vi "Distancias_ejes_convoy.vi"(2 "Series_flota1":string[](array[string]), 3 "Ejes_UT":i32[](array[numeric]), 4 "Puntos medios de las ventanas":dbl[][](array[numeric]), 5 "Series_flota":string[](array[string])) -> (1 "Distancias_entre_ejes_convoy":dbl[](array[numeric]))   [LabVIEW 2015]
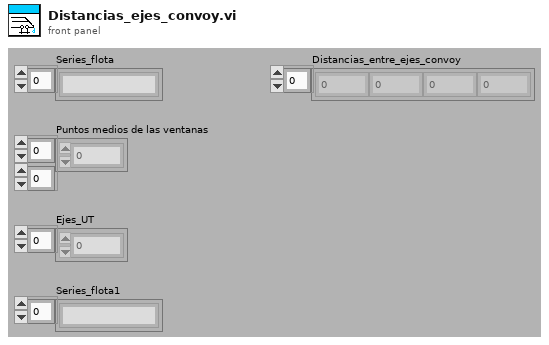
[diagram p1: front panel]
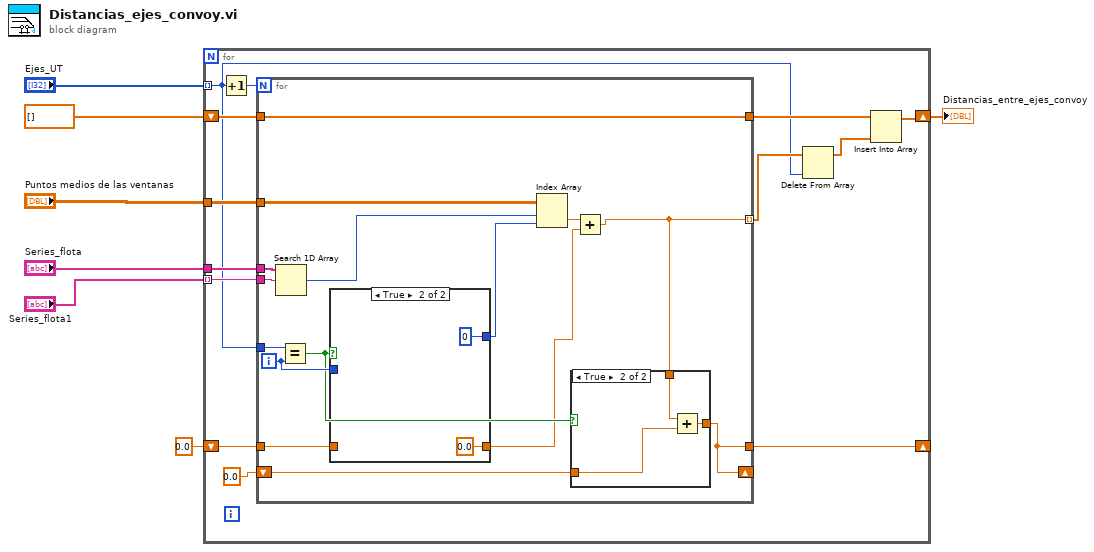
[diagram p0: block diagram]
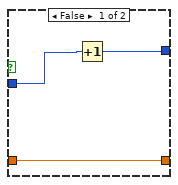
[diagram p3: hidden frame]
diagram:
  n1 = for {
    tunnel: "Puntos medios de las ventanas" -> [w20]
    tunnel: "Ejes_UT" -> [w11] mode=indexing
    tunnel: "Series_flota" -> [w18]
    tunnel: "Series_flota1" -> [w17] mode=indexing
    shift-right: [w14] -> w5
    shift-left: dbl[] [] -> [w16]
    shift-right: [w8] -> _
    shift-left: 0.0 -> [w9]
    n2 = Increment(x=w11) -> (x+1=w19:i32)
    n3 = for {
      N: w19 -> [_]
      tunnel: w20 -> [w30]
      tunnel: w11 -> [w33]
      tunnel: w18 -> [w32]
      tunnel: w17 -> [w31]
      tunnel: [w26] -> w13 mode=indexing
      tunnel: w16 -> [w28]
      tunnel: [w28] -> w15
      shift-right: [w24] -> _
      shift-left: 0.0 -> [w27]
      tunnel: w9 -> [w22]
      tunnel: [w24] -> w8
      i -> [w35]
      n4 = Search 1D Array(1D array=w32, element=w31) -> (index of element=w29:i32)  [unwired: 1 in]
      n5 = Equal?(x=w33, y=w35) -> (x = y?=w25:bool)
      n6 = case shown="True" w25 {
        tunnel: w35 -> [w42 _]
        tunnel: [w41 0] -> w34
        tunnel: w22 -> [w40 _]
        tunnel: [w40 0.0] -> w21
        frame False {
          n7 = Increment(x=w42) -> (x+1=w41:i32)
        }
        frame True {
        }
      }
      n8 = Index Array(array=w30, index (row)=w29, index (col)=w34) -> (element=w23:dbl)
      n9 = Add(x=w23, y=w21) -> (x+y=w26:dbl)
      n10 = case shown="True" w25 {
        tunnel: [w36 w38] -> w24
        tunnel: w26 -> [w36 w39]
        tunnel: w27 -> [_ w37]
        frame False {
        }
        frame True {
          n11 = Add(x=w39, y=w37) -> (x+y=w38:dbl)
        }
      }
    }
    n12 = Delete From Array(array=w13, index=w11) -> (array with subset deleted=w12:dbl[])  [unwired: 1 in, 1 out]
    n13 = Insert Into Array(array=w15, new element=w12) -> (w14:dbl[])  [unwired: 1 in]
  }
  "Distancias_entre_ejes_convoy" <- w5
